vi "FPGA Control.vi"() -> ()   [LabVIEW 2025]
uses:
  <vilib>/eio/EIONode/EIONode.xnode
  <vilib>/rvi/eio/common/nirviEmuTemplateMethod_errors.vi
panel:
  in  "Stop Control":bool
  out "Control Loop Rate (ticks)":u32
  out "Control Feedback":fxp<+/-,20,5>
  in  "Control Output":fxp<+/-,20,5>
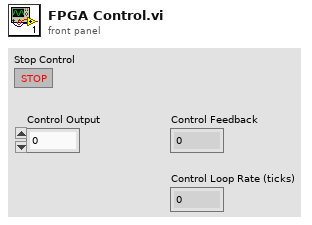
[diagram p1: front panel]
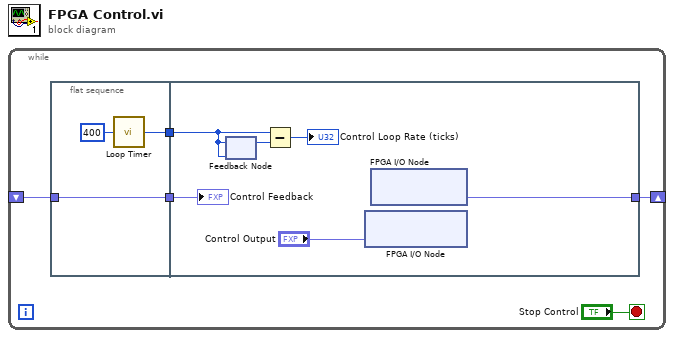
[diagram p0: block diagram]
diagram:
  n1 = while {
    shift-right: [w5] -> _
    shift-left: _ -> [w4]
    stop <- "Stop Control" stop-if-true
    n2 = flat-sequence {
      tunnel: w4 -> [w8]
      tunnel: [w8] -> w3
      tunnel: [w7] -> w2
      tunnel: [w14] -> w5
      tunnel: w3 -> [w9]
      tunnel: w2 -> [w12]
      frame #0 {
        n3 = call "Loop Timer"("Count(Ticks)"=u32 400) -> ("Tick Count(Ticks)"=w7:u32)
      }
      frame #1 {
        n4 = feedback-in #1(w12) -> ()
        n5 = feedback #1(w12) -> (w13:u32)
        n6 = Subtract(x=w12, y=w13) -> (x-y=→"Control Loop Rate (ticks)":u32)
        n7 = xnode "FPGA I/O Node"("Mod3/AO0"="Control Output") -> ()  [unwired: 1 in, 1 out]
        n8 = xnode "FPGA I/O Node"() -> ("Mod5/AI0"=w14:fxp<+/-,20,5>)  [unwired: 1 in, 1 out]
        "Control Feedback" <- w9
      }
    }
  }
